vi "OP Dash Send Values.vi"(10 "Robot Commands":T1) -> ()   [LabVIEW 2015]
uses:
  Robot Commands 2016.ctl
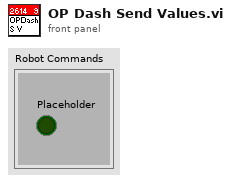
[diagram p1: front panel]
types:
  T1 = typedef "Robot Commands 2016.ctl" = cluster{"Placeholder":bool}
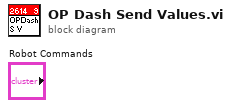
[diagram p0: block diagram]
diagram:
